vi "LUT.hot-cold4.vi"() -> (0 "Palette":cluster{u8, u8, u8}[](array[cluster]))   [LabVIEW 2013]
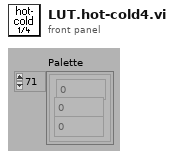
[diagram p1: front panel]
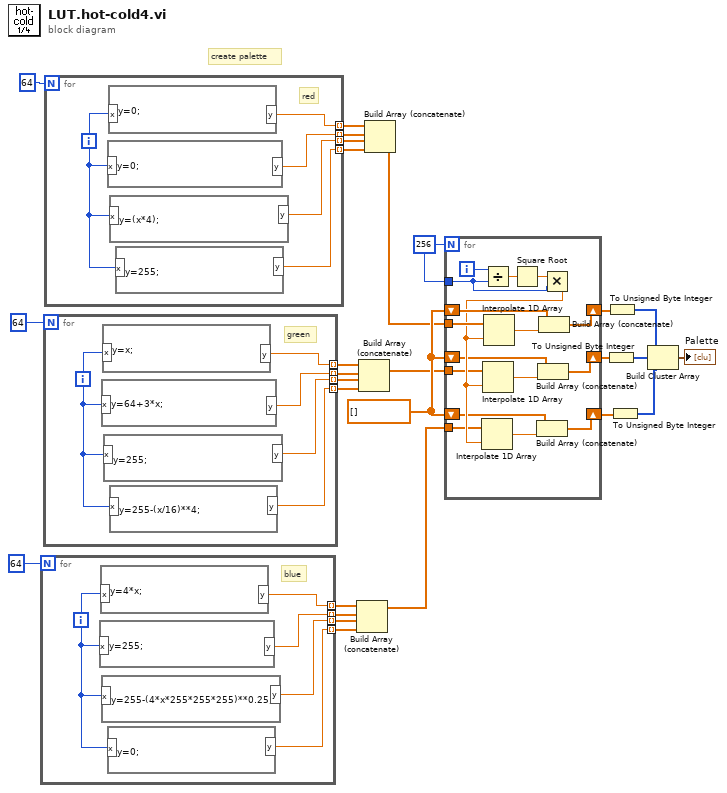
[diagram p0: block diagram]
diagram:
  w10 = dbl[] []
  w11 = 256
  # "create palette"
  n1 = for {
    N: 64 -> [_]
    tunnel: [w32] -> w16 mode=indexing
    tunnel: [w31] -> w15 mode=indexing
    tunnel: [w30] -> w14 mode=indexing
    tunnel: [w29] -> w13 mode=indexing
    i -> [w28]
    # "blue"
    n2 = formula code="y=255;"("x"=w28) -> ("y"=w31:dbl)
    n3 = formula code="y=4*x;"("x"=w28) -> ("y"=w32:dbl)
    n4 = formula code="y=255-(4*x*255*255*255)**0.25;"("x"=w28) -> ("y"=w30:dbl)
    n5 = formula code="y=0;"("x"=w28) -> ("y"=w29:dbl)
  }
  n6 = for {
    N: 64 -> [_]
    tunnel: [w37] -> w21 mode=indexing
    tunnel: [w36] -> w20 mode=indexing
    tunnel: [w35] -> w19 mode=indexing
    tunnel: [w34] -> w18 mode=indexing
    i -> [w33]
    # "green"
    n7 = formula code="y=64+3*x;"("x"=w33) -> ("y"=w36:dbl)
    n8 = formula code="y=x;"("x"=w33) -> ("y"=w37:dbl)
    n9 = formula code="y=255;"("x"=w33) -> ("y"=w35:dbl)
    n10 = formula code="y=255-(x/16)**4;"("x"=w33) -> ("y"=w34:dbl)
  }
  n11 = for {
    N: 64 -> [_]
    tunnel: [w42] -> w26 mode=indexing
    tunnel: [w41] -> w25 mode=indexing
    tunnel: [w40] -> w24 mode=indexing
    tunnel: [w39] -> w23 mode=indexing
    i -> [w38]
    # "red"
    n12 = formula code="y=0;"("x"=w38) -> ("y"=w41:dbl)
    n13 = formula code="y=0;"("x"=w38) -> ("y"=w42:dbl)
    n14 = formula code="y=(x*4);"("x"=w38) -> ("y"=w40:dbl)
    n15 = formula code="y=255;"("x"=w38) -> ("y"=w39:dbl)
  }
  n16 = Build Array (concatenate)(w16, w15, w14, w13) -> (w1:dbl[])
  n17 = Build Array (concatenate)(w21, w20, w19, w18) -> (w2:dbl[])
  n18 = Build Array (concatenate)(w26, w25, w24, w23) -> (w3:dbl[])
  n19 = for {
    N: w11 -> [_]
    tunnel: w11 -> [w58]
    tunnel: w3 -> [w57]
    shift-right: [w56] -> w9
    shift-left: w10 -> [w55]
    tunnel: w1 -> [w49]
    tunnel: w2 -> [w50]
    shift-right: [w45] -> w8
    shift-left: w10 -> [w48]
    shift-right: [w46] -> w7
    shift-left: w10 -> [w47]
    i -> [w59]
    n20 = Divide(x=w59, y=w58) -> (x/y=w44:dbl)
    n21 = Square Root(x=w44) -> (sqrt(x)=w43:dbl)
    n22 = Multiply(x=w43, y=w58) -> (x*y=w51:dbl)
    n23 = Interpolate 1D Array(1:w51, 2:w49) -> (0:w52:dbl)
    n24 = Interpolate 1D Array(1:w51, 2:w50) -> (0:w53:dbl)
    n25 = Interpolate 1D Array(1:w51, 2:w57) -> (0:w54:dbl)
    n26 = Build Array (concatenate)(w47, w52) -> (w46:dbl[])
    n27 = Build Array (concatenate)(w48, w53) -> (w45:dbl[])
    n28 = Build Array (concatenate)(w55, w54) -> (w56:dbl[])
  }
  n29 = To Unsigned Byte Integer(number=w8) -> (unsigned 8bit integer=w5:u8[])
  n30 = To Unsigned Byte Integer(number=w9) -> (unsigned 8bit integer=w4:u8[])
  n31 = To Unsigned Byte Integer(number=w7) -> (unsigned 8bit integer=w6:u8[])
  n32 = Build Cluster Array(w4, w5, w6) -> (→"Palette":cluster{u8, u8, u8}[])
